vi "AD5933_ImpedanceConversion (SubVI).vi"(5 "Measurement Raw Data":T1) -> (0 "Phase":dbl[](array[numeric]), 1 "Impedance":dbl[](array[numeric]), 2 "Imaginary Part":dbl[](array[numeric]), 3 "Real Part":dbl[](array[numeric]), 4 "Temperature":dbl)   [LabVIEW 2017]
uses:
  TypeDefs/MeasurementRawData.ctl
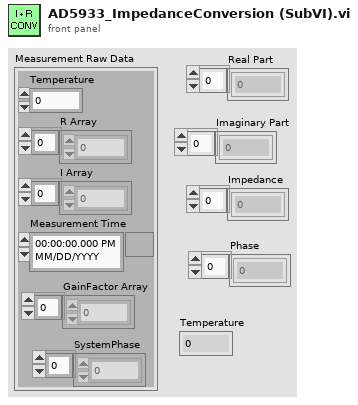
[diagram p1: front panel]
types:
  T1 = typedef "MeasurementRawData.ctl" = cluster{"Temperature":dbl, "R Array":dbl[], "I Array":dbl[], "Measurement Time":timestamp, "GainFactor Array":dbl[], "SystemPhase":dbl[]}
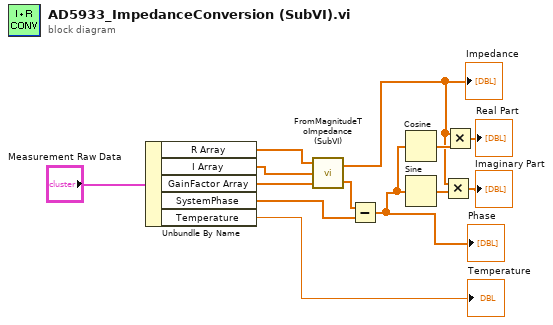
[diagram p0: block diagram]
diagram:
  n1 = Unbundle By Name("Measurement Raw Data") -> ("R Array"=w10:dbl[], "I Array"=w11:dbl[], "GainFactor Array"=w12:dbl[], "SystemPhase"=w9:dbl[], "Temperature"=→"Temperature":dbl)
  n2 = call "FromMagnitudeToImpedance (SubVI).vi"("GainFactor"=w12, "I"=w11, "R"=w10) -> ("Phase"=w5:dbl[], "Impedance"=w4:dbl[])
  "Impedance" <- w4
  n3 = Subtract(x=w5, y=w9) -> (x-y=w1:dbl[])
  "Phase" <- w1
  n4 = Cosine(x=w1) -> (cos(x)=w7:dbl[])
  n5 = Sine(x=w1) -> (sin(x)=w6:dbl[])
  n6 = Multiply(x=w4, y=w6) -> (x*y=→"Imaginary Part":dbl[])
  n7 = Multiply(x=w4, y=w7) -> (x*y=→"Real Part":dbl[])
